vi "Reference Imaging Source.vi"() -> ()   [LabVIEW 2014]
uses:
  <vilib>/userdefined/High Color/IMAQdx.ctl
  <vilib>/vision/driver/IMAQdx.llb/IMAQdx Buffer Number Mode.ctl
  <vilib>/vision/driver/NI_Vision_Acquisition_Software.lvlib
  <resource>/objmgr/imaqdx.rc
panel:
  out "Ref Path":path
  out "Init Message":string
  out "Device Serial Number":string
  out "Success?":bool
  out "error out  - closing camera":errorcluster
  out "Message":string
  out "Warning":bool
  in  "Overwrite?":bool
  in  "Exposure Time µs":dbl=50.0 min=50.0 max=2000000.0 step=1.0 format="%#_8f"
  out "Buffer Number Out":u32
  in  "Nom Ref":string="ref"
  in  "File Path (for Snap! function)":path
  in  "snap":bool
  in  "Gain (dB)":dbl=18.06 min=0.0 max=18.06 step=0.1
  in  "File to ref":bool
  in  "Ref To File":bool
  in  "End Point 2":cluster{"X":i32, "Y":i32}
  in  "Start Point 2":cluster{"X":i32, "Y":i32}
  in  "End Point 1":cluster{"X":i32, "Y":i32}
  in  "Start Point 1":cluster{"X":i32, "Y":i32}
  out "error out":errorcluster
  in  "error in (no error)":errorcluster
  in  "Rectangle d'encardrement":T1
  in  "ref":bool
  out "Coordonnées":i32[](array[numeric])
  in  "stop":bool
  out "Image":T2(plugin-control)
  in  "Session":T3="cam0"
  # "Références Champs Proches/Champs Lointains"
  # "Utiliser outil OVALE pour effectuer la sélection"
  # "Beta version :)"
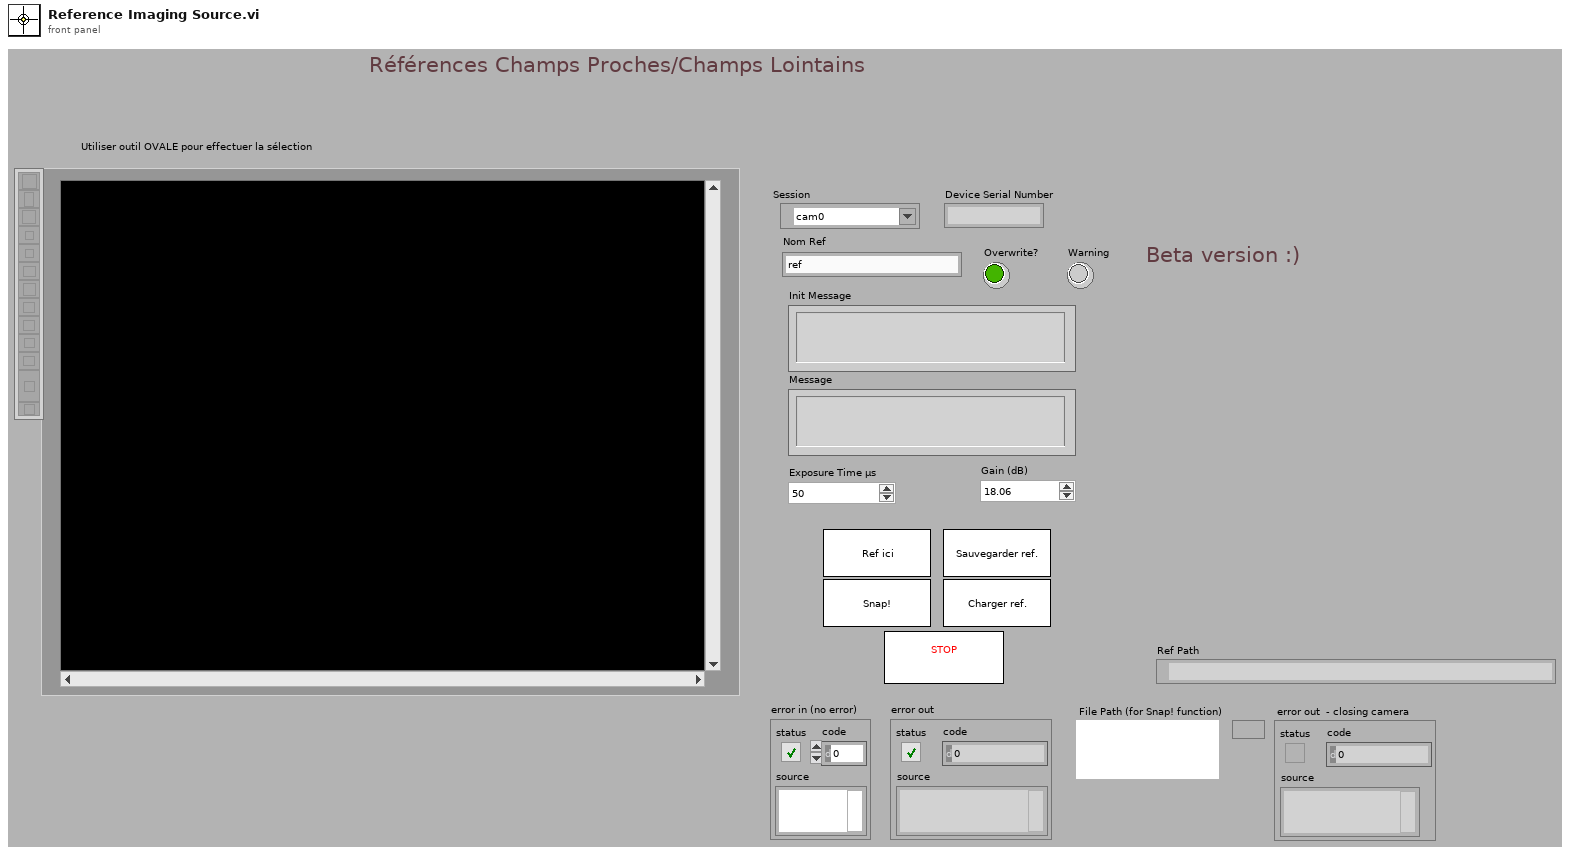
[diagram p1: front panel]
types:
  T1 = cluster{"Left":i32, "Top":i32, "Right":i32, "Bottom":i32}
  T2 = typedef "IMAQ Image.ctl" = refnum<image>
  T3 = typedef "IMAQdx.ctl" = refnum<k21>
  T4 = enum16{"open", "replace", "create", "open or create", "replace or create", "replace or create with confirmation"}
  T5 = typedef "NI_Vision_Acquisition_Software.lvlib/IMAQdx Buffer Number Mode.ctl" = enum32{"Next", "Last", "Buffer Number"}
  T6 = enum8{"Enabled", "Disabled", "Disabled and Grayed Out"}
  T7 = typedef "Image Type" = u32
  T8 = cluster{"Start Point 1":cluster{"X":i32, "Y":i32}, "End Point 1":cluster{"X":i32, "Y":i32}, "Start Point 2":cluster{"X":i32, "Y":i32}, "End Point 2":cluster{"X":i32, "Y":i32}}
  T9 = enum32{"invalid app kind", "Development System", "Run Time System", "Student Edition", "Embedded LabVIEW", "Evaluation", "Custom"}
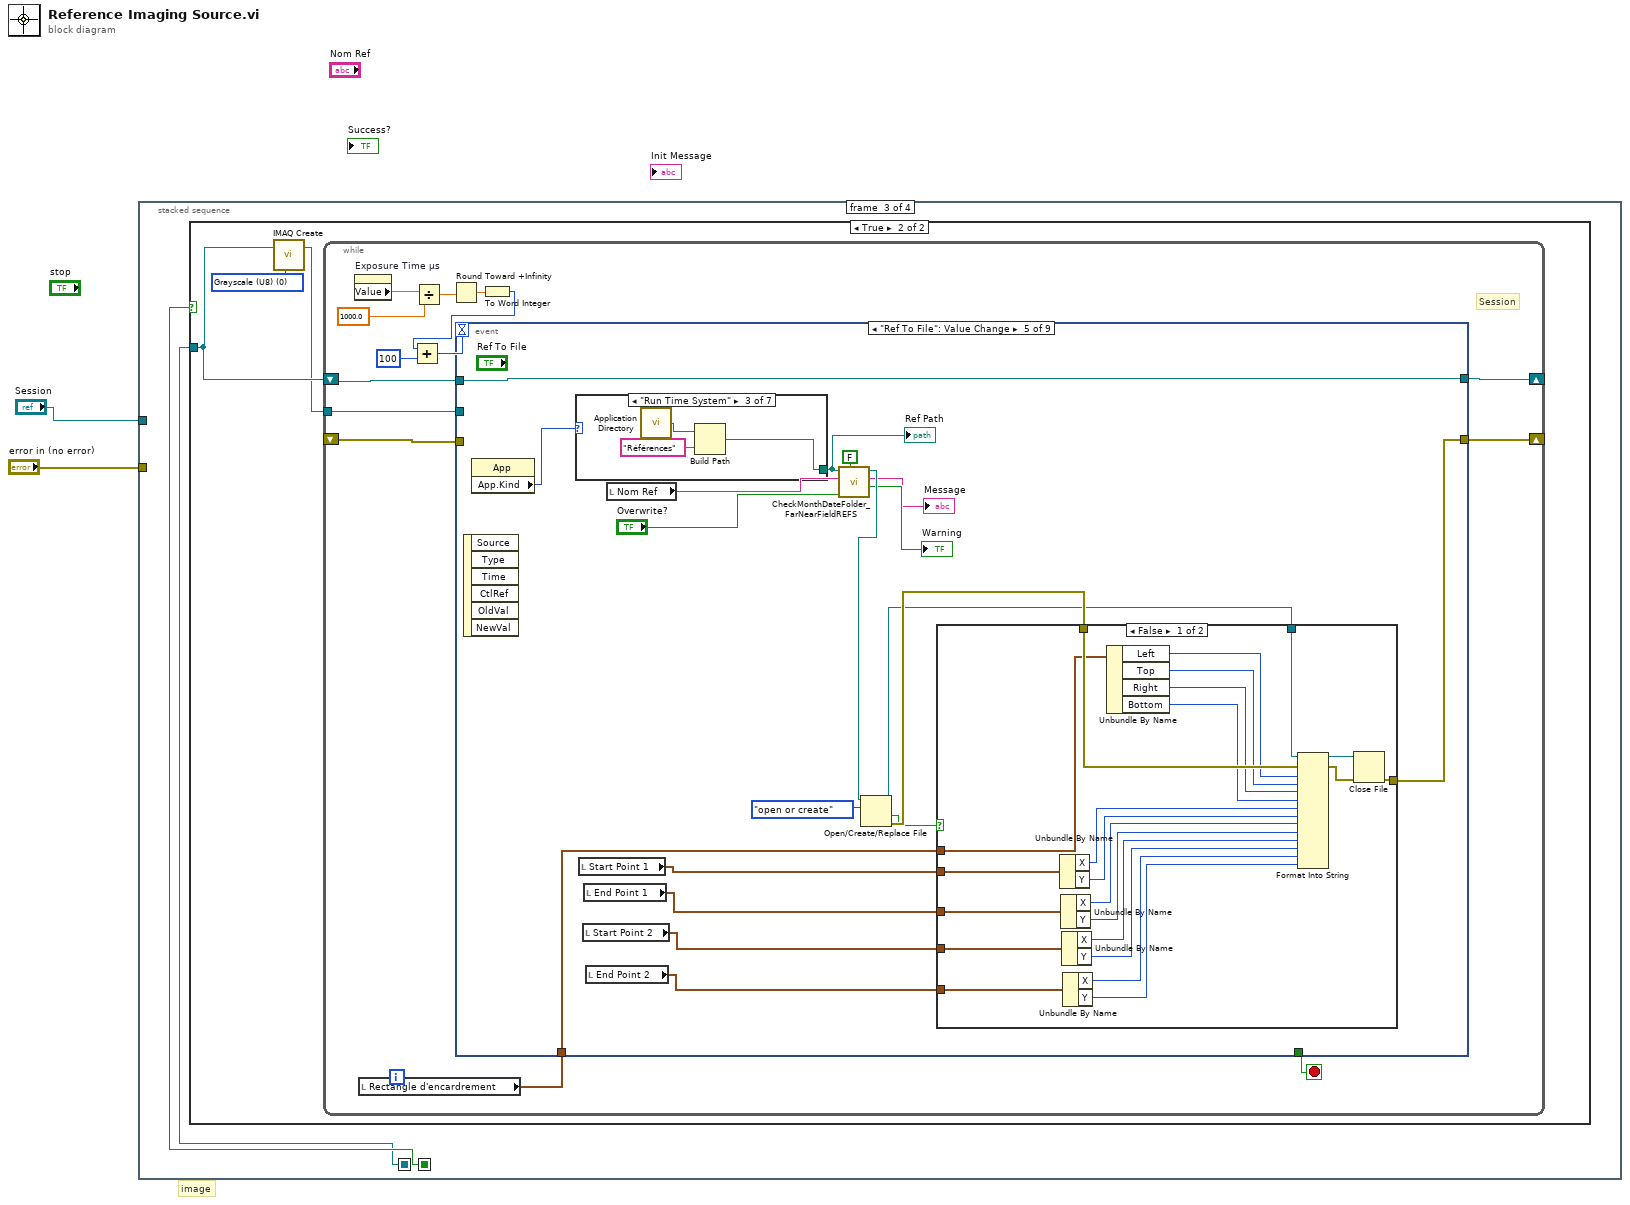
[diagram p0: block diagram]
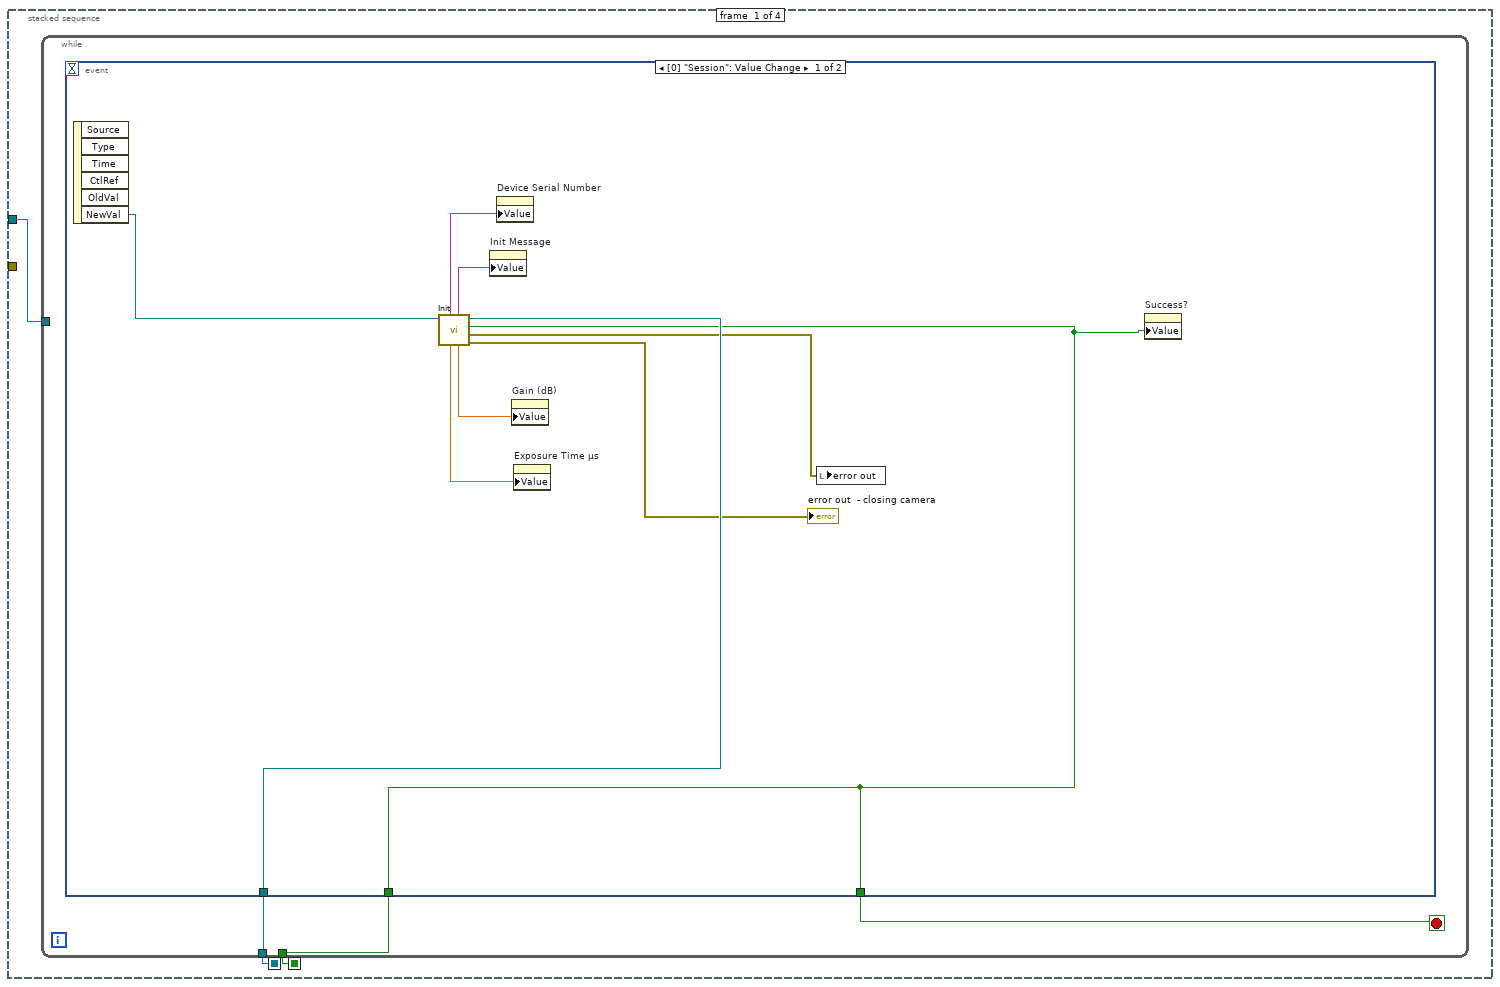
[diagram p2: hidden frame]
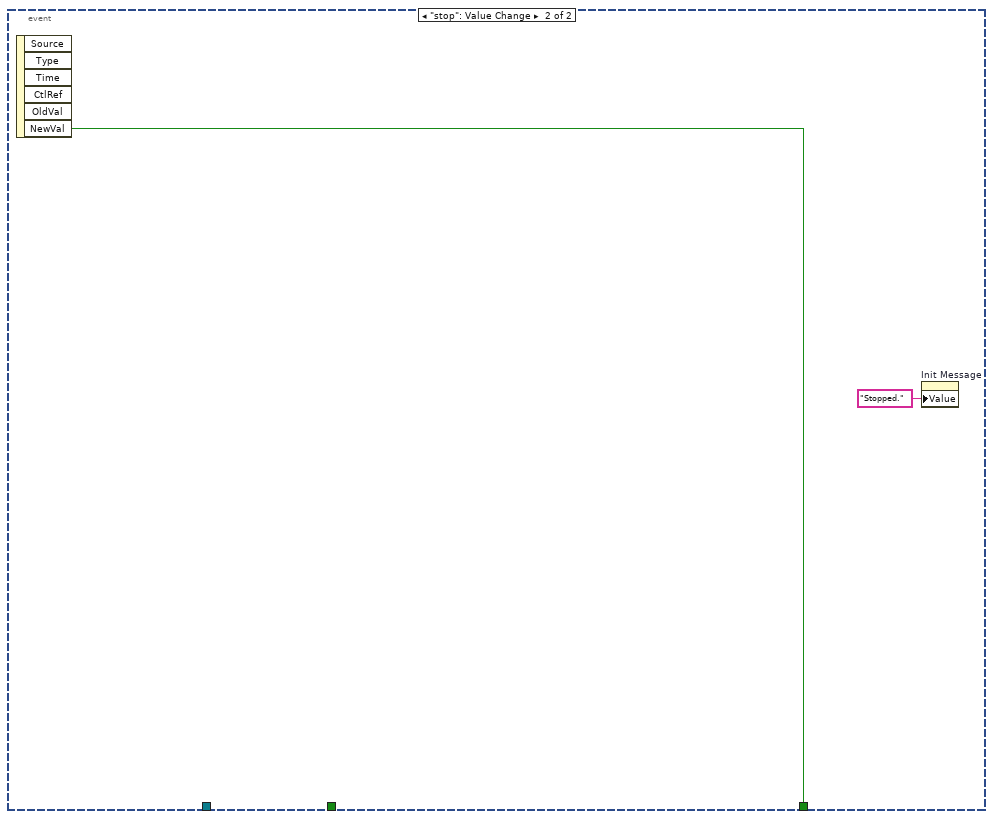
[diagram p3: hidden frame]
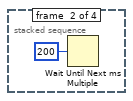
[diagram p4: hidden frame]
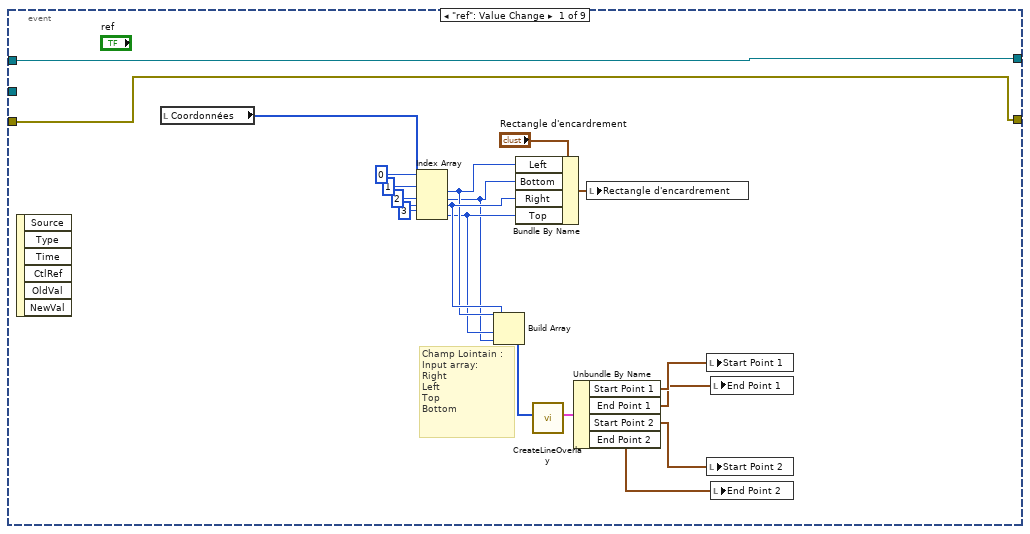
[diagram p6: hidden frame]
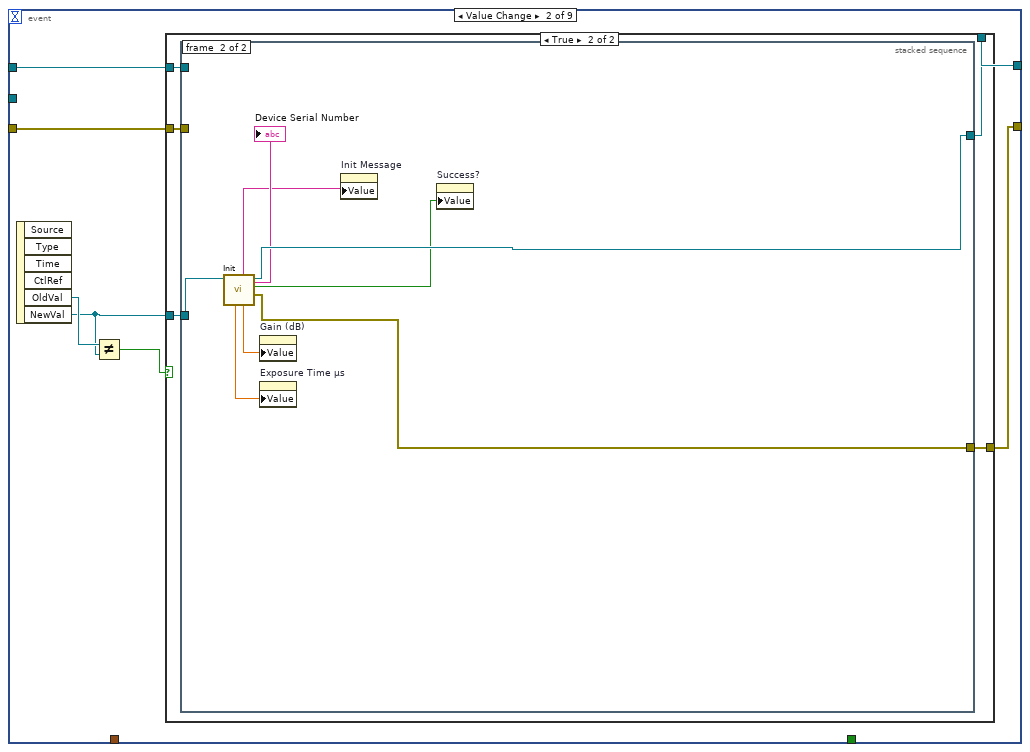
[diagram p7: hidden frame]
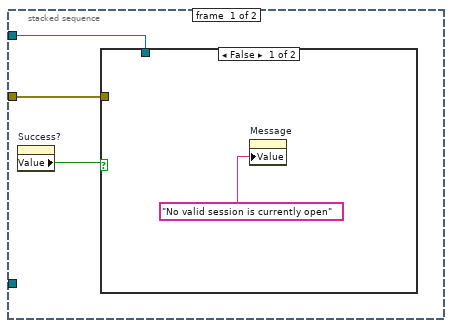
[diagram p9: hidden frame]
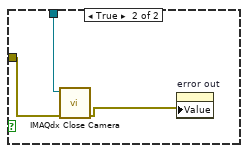
[diagram p10: hidden frame]
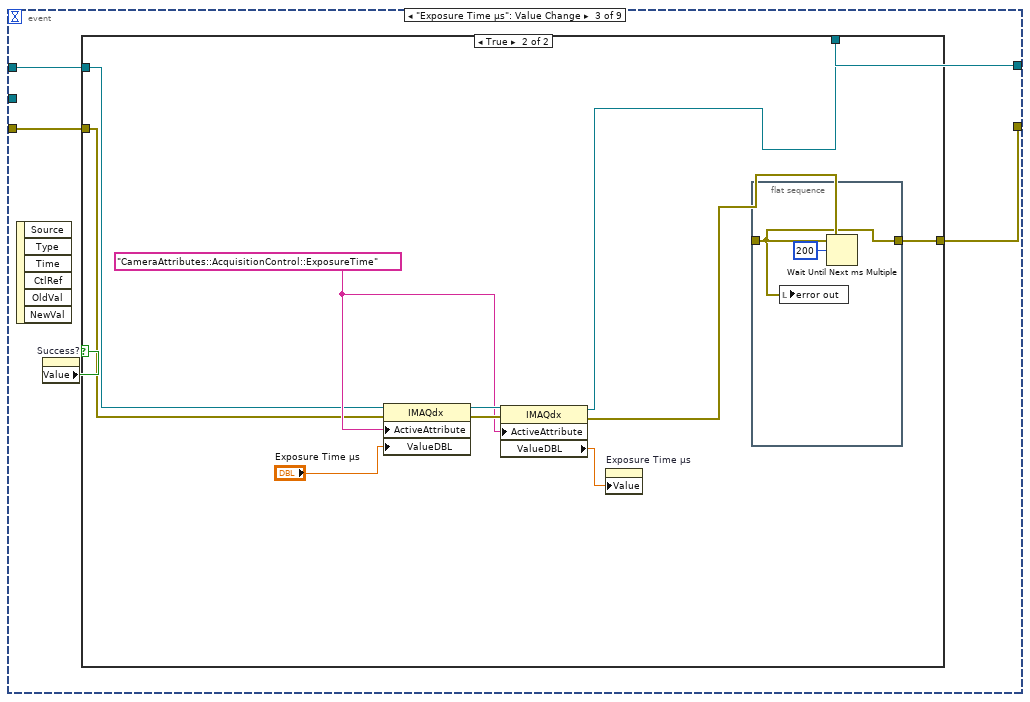
[diagram p11: hidden frame]
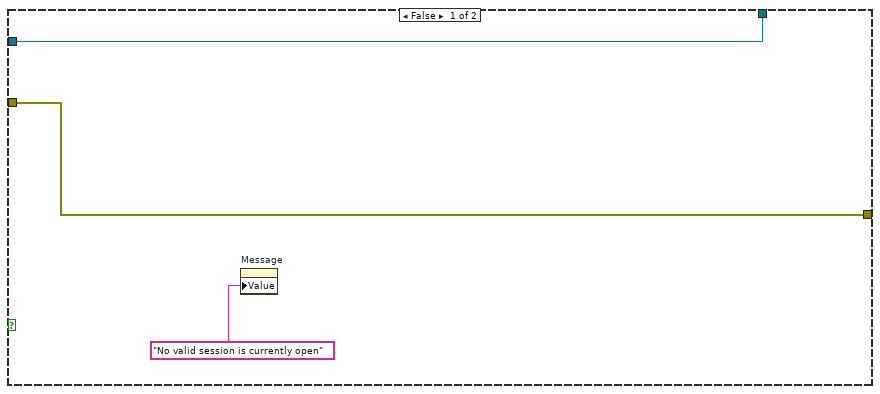
[diagram p12: hidden frame]
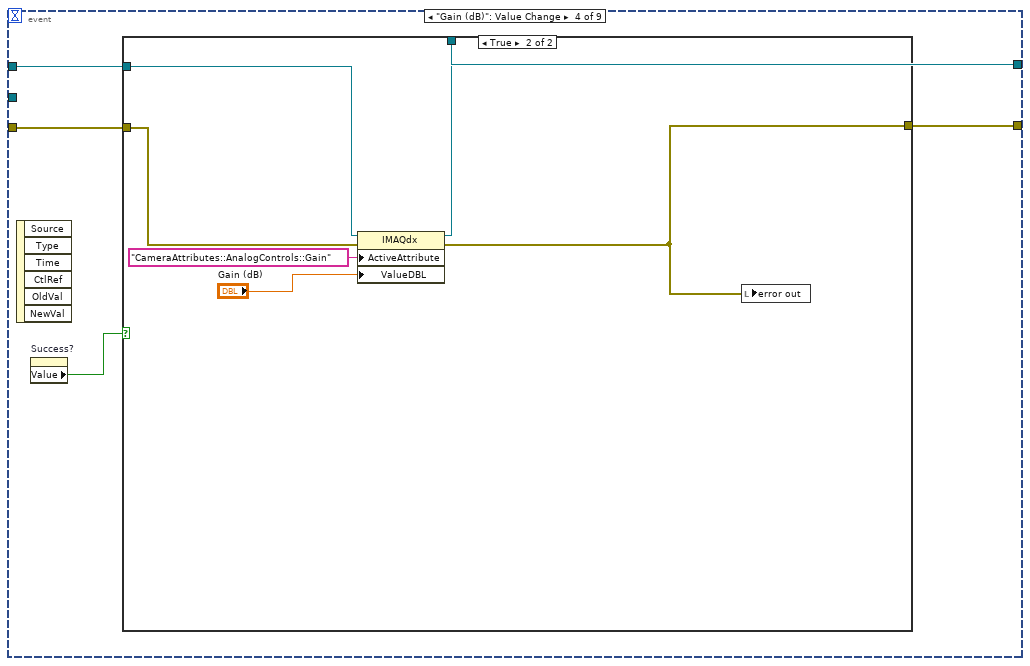
[diagram p13: hidden frame]
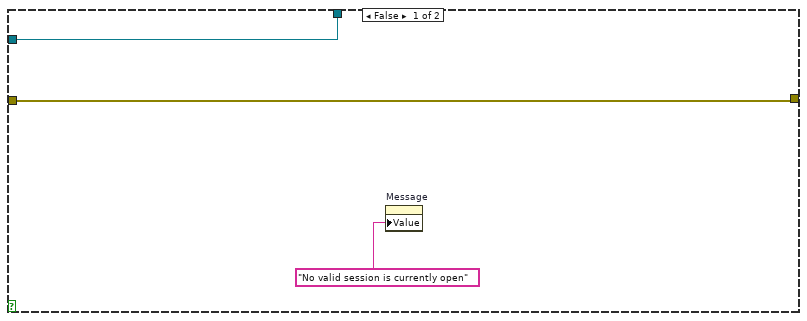
[diagram p14: hidden frame]
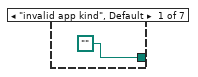
[diagram p15: hidden frame]
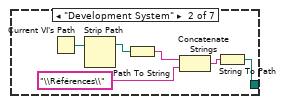
[diagram p16: hidden frame]
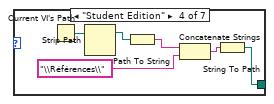
[diagram p17: hidden frame]
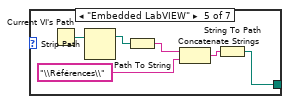
[diagram p18: hidden frame]
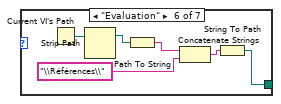
[diagram p19: hidden frame]
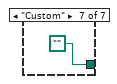
[diagram p20: hidden frame]
diagram:
  # "image"
  n1 = stacked-sequence {
    seq-local: [w4 _ _ _] -> [_ _ w21 _]
    seq-local: [w3 _ _ _] -> [_ _ w22 _]
    tunnel: "Session" -> [w5 _ _ _]
    tunnel: "error in (no error)" -> [_ _ _ _]
    frame #0 {
      n2 = while {
        tunnel: w5 -> [_]
        tunnel: [w7] -> w4
        tunnel: [w6] -> w3
        stop <- w8 stop-if-true
        n3 = event shown="[0] \"Session\": Value Change" {
          selector: _ -> [_ _]
          dyn-events: _ -> [_ _]
          timeout: _ -> [_ _]
          tunnel: [w9 w19] -> w8
          tunnel: [w17 _] -> w7
          tunnel: [w9 _] -> w6
          event Value Change {
            n4 = event-data() -> ("NewVal"=w16:T3)  [unwired: 1 in, 5 out]
            n5 = call "Init.vi"("Session"=w16) -> ("error out  - closing camera"=→"error out  - closing camera":errorcluster, "error out"=w13:errorcluster, "Success?"=w9:bool, "IMAQdx Session OUT"=w17:T3, "Gain - READ"=w15:dbl, "Message"=w11:string, "Exposure Time - READ"=w14:dbl, "Device Serial Number"=w10:string)  [unwired: 3 in]
            n6 = property on="Init Message" class="Str"("Value"=w11) -> ()  [unwired: 2 in, 2 out]
            n7 = property on="Device Serial Number" class="Str"("Value"=w10) -> ()  [unwired: 2 in, 2 out]
            n8 = property on="Gain (dB)" class="DigNum (strict)"("Value"=w15) -> ()  [unwired: 2 in, 2 out]
            n9 = property on="Exposure Time µs" class="DigNum (strict)"("Value"=w14) -> ()  [unwired: 2 in, 2 out]
            n10 = local write "error out"(w13) -> ()
            n11 = property on="Success?" class="Bool (strict)"("Value"=w9) -> ()  [unwired: 2 in, 2 out]
          }
          event "stop": Value Change {
            n12 = event-data() -> ("NewVal"=w19:bool)  [unwired: 1 in, 5 out]
            n13 = property on="Init Message" class="Str"("Value"="Stopped." ("Init Message")) -> ()  [unwired: 2 in, 2 out]
          }
        }
      }
    }
    frame #1 {
      n14 = Wait Until Next ms Multiple(millisecond multiple=u32 200) -> ()  [unwired: 1 out]
    }
    frame #2 {
      n15 = case shown="True" w22 {
        tunnel: w21 -> [_ w24]
        frame False {
        }
        frame True {
          w25 = T7 0 items=["Grayscale (U8)", "Grayscale (I16)", "Grayscale (SGL)", "Complex (CSG)", "RGB (U32)", "HSL (U32)", "RGB (U64)", "Grayscale (U16)"] ("Image Type")
          n16 = call "IMAQ Create"("Image Name"=w24, "Image Type"=w25) -> ("New Image"=w23:T2)  [unwired: 2 in, 2 out]
          n17 = while {
            shift-right: [w37] -> _
            shift-left: _ -> [w38]
            shift-right: [w35] -> _
            shift-left: w24 -> [w36]
            tunnel: w23 -> [w26]
            stop <- w39 stop-if-true
            # "Session"
            n18 = property on="Exposure Time µs" class="DigNum (strict)"() -> ("Value"=w27:dbl)  [unwired: 2 in, 2 out]
            n19 = local read "Rectangle d'encardrement"() -> (w28:T1)
            n20 = Divide(x=w27, y=1000.0) -> (x/y=w30:dbl)
            n21 = Round Toward +Infinity(x=w30) -> (ceil(x): smallest int >= x=w32:dbl)
            n22 = To Word Integer(number=w32) -> (16bit integer=w29:i16)
            n23 = Add(x=w29, y=i16 100) -> (x+y=w33:i16)
            n24 = event shown="[4] \"Ref To File\": Value Change" {
              selector: _ -> [_ _ _ _ _ _ _ _ _]
              dyn-events: _ -> [_ _ _ _ _ _ _ _ _]
              timeout: w33 -> [_ _ _ _ _ _ _ _ _]
              tunnel: [_ _ _ _ _ _ _ w254 _] -> w39
              tunnel: w38 -> [w40 w65 w90 w112 _ w203 w238 w255 w268]
              tunnel: [w40 w63 w92 w109 w136 w198 w239 _ w267] -> w37
              tunnel: w36 -> [w41 w62 w91 w111 w124 w197 w237 w256 w266]
              tunnel: [w41 w64 w89 w110 w124 w197 w236 _ w265] -> w35
              tunnel: w28 -> [_ _ _ _ w135 _ _ _ _]
              tunnel: w26 -> [_ _ _ _ _ _ w235 _ w260]
              event "ref": Value Change {
                # "Champ Lointain :\nInput array:\nRight\nLeft\nTop\nBottom"
                n25 = event-data() -> ()  [unwired: 1 in, 6 out]
                n26 = local read "Coordonnées"() -> (w52:i32[])
                n27 = Index Array(array=w52, index #1=0 ("index"), index #2=1 ("index"), index #3=2 ("index"), index #4=3 ("index")) -> (element #1=w45:i32, element #2=w43:i32, element #3=w46:i32, element #4=w44:i32)
                n28 = Build Array(w46, w45, w44, w43) -> (w42:i32[])
                n29 = Bundle By Name(cluster="Rectangle d'encardrement", "Left"=w45, "Bottom"=w43, "Right"=w46, "Top"=w44) -> (w53:T1)
                n30 = call "CreateLineOverlay.vi"("Bounding rectangle"=w42) -> ("Lines"=w51:T8)  [unwired: 8 in, 1 out]
                n31 = Unbundle By Name(w51) -> ("Start Point 1"=w50:cluster{"X":i32, "Y":i32}, "End Point 1"=w49:cluster{"X":i32, "Y":i32}, "Start Point 2"=w48:cluster{"X":i32, "Y":i32}, "End Point 2"=w47:cluster{"X":i32, "Y":i32})
                n32 = local write "Rectangle d'encardrement"(w53) -> ()
                n33 = local write "Start Point 1"(w50) -> ()
                n34 = local write "Start Point 2"(w48) -> ()
                n35 = local write "End Point 1"(w49) -> ()
                n36 = local write "End Point 2"(w47) -> ()
              }
              event Value Change {
                n37 = event-data() -> ("OldVal"=w60:T3, "NewVal"=w59:T3)  [unwired: 1 in, 4 out]
                n38 = Not Equal?(x=w60, y=w59) -> (x != y?=w61:bool)
                n39 = case shown="True" w61 {
                  tunnel: w65 -> [w66 w72]
                  tunnel: w59 -> [w67 w71]
                  tunnel: [w67 w70] -> w64
                  tunnel: [w66 w69] -> w63
                  tunnel: w62 -> [_ w68]
                  frame False {
                  }
                  frame True {
                    n40 = stacked-sequence {
                      tunnel: w72 -> [w75 _]
                      tunnel: w71 -> [_ w87]
                      tunnel: [_ w84] -> w70
                      tunnel: [_ w82] -> w69
                      tunnel: w68 -> [w74 _]
                      frame #0 {
                        n41 = property on="Success?" class="Bool (strict)"() -> ("Value"=w73:bool)  [unwired: 2 in, 2 out]
                        n42 = case shown="False" w73 {
                          tunnel: w75 -> [_ w79]
                          tunnel: w74 -> [_ w77]
                          frame False {
                            n43 = property on="Message" class="Str"("Value"="No valid session is currently open" ("Message")) -> ()  [unwired: 2 in, 2 out]
                          }
                          frame True {
                            n44 = call <vilib>:"IMAQdx Close Camera.vi"("error in"=w79, "Session In"=w77) -> ("error out"=w78:errorcluster)  [unwired: 9 in]
                            n45 = property on="error out" class="Clust (strict)"("Value"=w78) -> ()  [unwired: 2 in, 2 out]
                          }
                        }
                      }
                      frame #1 {
                        n46 = call "Init.vi"("Session"=w87) -> ("error out"=w82:errorcluster, "Success?"=w83:bool, "IMAQdx Session OUT"=w84:T3, "Gain - READ"=w86:dbl, "Message"=w80:string, "Exposure Time - READ"=w85:dbl, "Device Serial Number"=→"Device Serial Number":string)  [unwired: 3 in, 1 out]
                        n47 = property on="Gain (dB)" class="DigNum (strict)"("Value"=w86) -> ()  [unwired: 2 in, 2 out]
                        n48 = property on="Exposure Time µs" class="DigNum (strict)"("Value"=w85) -> ()  [unwired: 2 in, 2 out]
                        n49 = property on="Init Message" class="Str"("Value"=w80) -> ()  [unwired: 2 in, 2 out]
                        n50 = property on="Success?" class="Bool (strict)"("Value"=w83) -> ()  [unwired: 2 in, 2 out]
                      }
                    }
                  }
                }
              }
              event "Exposure Time µs": Value Change {
                n51 = event-data() -> ()  [unwired: 1 in, 6 out]
                n52 = property on="Success?" class="Bool (strict)"() -> ("Value"=w88:bool)  [unwired: 2 in, 2 out]
                n53 = case shown="True" w88 {
                  tunnel: [w94 w104] -> w92
                  tunnel: w91 -> [w95 w96]
                  tunnel: w90 -> [w94 w97]
                  tunnel: [w95 w101] -> w89
                  frame False {
                    n54 = property on="Message" class="Str"("Value"="No valid session is currently open" ("Message")) -> ()  [unwired: 2 in, 2 out]
                  }
                  frame True {
                    w98 = "CameraAttributes::AcquisitionControl::ExposureTime" ("ActiveAttribute")
                    n55 = property class="IMAQdx"(reference=w96, error in=w97, "ActiveAttribute"=w98, "ValueDBL"="Exposure Time µs") -> (reference out=w103:T3, error out=w102:errorcluster)
                    n56 = property class="IMAQdx"(reference=w103, error in=w102, "ActiveAttribute"=w98) -> (reference out=w101:T3, error out=w100:errorcluster, "ValueDBL"=w99:dbl)
                    n57 = property on="Exposure Time µs" class="DigNum (strict)"("Value"=w99) -> ()  [unwired: 2 in, 2 out]
                    n58 = flat-sequence {
                      tunnel: w100 -> [w106]
                      tunnel: [w106] -> w104
                      frame #0 {
                        n59 = local write "error out"(w106) -> ()
                        n60 = Wait Until Next ms Multiple(millisecond multiple=u32 200) -> ()  [unwired: 1 out]
                      }
                    }
                  }
                }
              }
              event "Gain (dB)": Value Change {
                n61 = event-data() -> ()  [unwired: 1 in, 6 out]
                n62 = property on="Success?" class="Bool (strict)"() -> ("Value"=w108:bool)  [unwired: 2 in, 2 out]
                n63 = case shown="True" w108 {
                  tunnel: w112 -> [w115 w121]
                  tunnel: w111 -> [w114 w118]
                  tunnel: [w114 w117] -> w110
                  tunnel: [w115 w116] -> w109
                  frame False {
                    n64 = property on="Message" class="Str"("Value"="No valid session is currently open" ("Message")) -> ()  [unwired: 2 in, 2 out]
                  }
                  frame True {
                    n65 = property class="IMAQdx"(reference=w118, error in=w121, "ActiveAttribute"="CameraAttributes::AnalogControls::Gain", "ValueDBL"="Gain (dB)") -> (reference out=w117:T3, error out=w116:errorcluster)
                    n66 = local write "error out"(w116) -> ()
                  }
                }
              }
              event "Ref To File": Value Change {
                n67 = event-data() -> ()  [unwired: 1 in, 6 out]
                n68 = property class="App"() -> ("App.Kind"=w123:T9)  [unwired: 2 in, 2 out]
                n69 = case shown="\"Run Time System\"" w123 {
                  tunnel: [path "" w142 w148 w151 w157 w163 path ""] -> w130
                  frame "invalid app kind", Default {
                  }
                  frame "Development System" {
                    n70 = Current VI's Path() -> (path=w147:path)
                    n71 = Strip Path(path=w147) -> (stripped path=w146:path)  [unwired: 1 out]
                    n72 = Path To String(path=w146) -> (string=w145:string)
                    n73 = Concatenate Strings(w145, "\\Références\\") -> (w143:string)
                    n74 = String To Path(string=w143) -> (path=w142:path)
                  }
                  frame "Run Time System" {
                    n75 = call <vilib>:"Application Directory.vi"() -> ("Application Directory"=w150:path)
                    n76 = Build Path(base path=w150, name or relative path="Références") -> (appended path=w148:path)
                  }
                  frame "Student Edition" {
                    n77 = Current VI's Path() -> (path=w156:path)
                    n78 = Strip Path(path=w156) -> (stripped path=w155:path)  [unwired: 1 out]
                    n79 = Path To String(path=w155) -> (string=w154:string)
                    n80 = Concatenate Strings(w154, "\\Références\\") -> (w152:string)
                    n81 = String To Path(string=w152) -> (path=w151:path)
                  }
                  frame "Embedded LabVIEW" {
                    n82 = Current VI's Path() -> (path=w162:path)
                    n83 = Strip Path(path=w162) -> (stripped path=w161:path)  [unwired: 1 out]
                    n84 = Path To String(path=w161) -> (string=w160:string)
                    n85 = Concatenate Strings(w160, "\\Références\\") -> (w158:string)
                    n86 = String To Path(string=w158) -> (path=w157:path)
                  }
                  frame "Evaluation" {
                    n87 = Current VI's Path() -> (path=w168:path)
                    n88 = Strip Path(path=w168) -> (stripped path=w167:path)  [unwired: 1 out]
                    n89 = Path To String(path=w167) -> (string=w166:string)
                    n90 = Concatenate Strings(w166, "\\Références\\") -> (w164:string)
                    n91 = String To Path(string=w164) -> (path=w163:path)
                  }
                  frame "Custom" {
                  }
                }
                "Ref Path" <- w130
                n92 = local read "Start Point 1"() -> (w134:cluster{"X":i32, "Y":i32})
                n93 = local read "Start Point 2"() -> (w132:cluster{"X":i32, "Y":i32})
                n94 = local read "End Point 1"() -> (w133:cluster{"X":i32, "Y":i32})
                n95 = local read "End Point 2"() -> (w131:cluster{"X":i32, "Y":i32})
                n96 = local read "Nom Ref"() -> (w129:string)
                n97 = call "CheckMonthDateFolder_FarNearFieldREFS.vi"("Folder Path Control"=w130, "File Name"=w129, "Overwrite?"="Overwrite?", "Automatic date folder nesting?"=FALSE) -> ("File Path"=w127:path, "Message"=→"Message":string, "Warning"=→"Warning":bool)  [unwired: 4 in]
                n98 = Open/Create/Replace File(file path (use dialog)=w127, operation (0:open)=T4."open or create") -> (refnum out=w138:refnum<file>, cancelled=w137:bool, error out=w139:errorcluster)  [unwired: 4 in]
                n99 = case shown="False" w137 {
                  tunnel: w139 -> [w191 w196]
                  tunnel: w138 -> [w189 _]
                  tunnel: [w175 w192] -> w136
                  tunnel: w135 -> [w174 _]
                  tunnel: w134 -> [w173 _]
                  tunnel: w133 -> [w172 _]
                  tunnel: w132 -> [w171 _]
                  tunnel: w131 -> [w170 _]
                  frame False {
                    n100 = Unbundle By Name(w173) -> ("X"=w185:i32, "Y"=w184:i32)
                    n101 = Unbundle By Name(w172) -> ("X"=w183:i32, "Y"=w182:i32)
                    n102 = Unbundle By Name(w171) -> ("X"=w181:i32, "Y"=w180:i32)
                    n103 = Unbundle By Name(w170) -> ("X"=w179:i32, "Y"=w178:i32)
                    n104 = Unbundle By Name(w174) -> ("Left"=w190:i32, "Top"=w188:i32, "Right"=w187:i32, "Bottom"=w186:i32)
                    n105 = Format Into String(initial string=w189, error in=w191, w190, w188, w187, w186, w185, w184, w183, w182, w181, w180, w179, w178) -> (resulting string=w177:refnum<file>, error out=w176:errorcluster)  [unwired: 1 in]
                    n106 = Close File(refnum=w177, error in=w176) -> (error out=w175:errorcluster)  [unwired: 1 out]
                  }
                  frame True {
                    n107 = Bundle By Name(cluster=w196, "status"=FALSE, "code"=0, "source"="") -> (w192:errorcluster)
                  }
                }
              }
              event "File to ref": Value Change {
                n108 = event-data() -> ()  [unwired: 1 in, 6 out]
                n109 = Open/Create/Replace File(error in=w203, prompt="Fichier à charger", access (0:read/write)=enum16{"read/write", "read-only", "write-only"}."read-only") -> (refnum out=w200:refnum<file>, cancelled=w199:bool, error out=w202:errorcluster)  [unwired: 3 in]
                n110 = case shown="False" w199 {
                  tunnel: w202 -> [w208 _]
                  tunnel: w200 -> [w231 _]
                  tunnel: [w205 errorcluster {"status"=FALSE, "code"=0, "source"=""} ("error out")] -> w198
                  frame False {
                    n111 = Scan From String("%d %d %d %d %d %d %d %d %d %d %d %d" ("format string"), w231, w208) -> (w207:refnum<file>, w206:errorcluster, output 1=w228:i32, output 2=w227:i32, output 3=w226:i32, output 4=w225:i32, output 5=w223:i32, output 6=w222:i32, output 7=w218:i32, output 8=w217:i32, output 9=w214:i32, output 10=w213:i32, output 11=w210:i32, output 12=w209:i32)  [unwired: 12 in]
                    n112 = local read "Rectangle d'encardrement"() -> (w230:T1)
                    n113 = local read "Start Point 2"() -> (w216:cluster{"X":i32, "Y":i32})
                    n114 = local read "End Point 2"() -> (w212:cluster{"X":i32, "Y":i32})
                    n115 = local read "Start Point 1"() -> (w224:cluster{"X":i32, "Y":i32})
                    n116 = local read "End Point 1"() -> (w220:cluster{"X":i32, "Y":i32})
                    n117 = Bundle By Name(cluster=w224, "X"=w223, "Y"=w222) -> (w221:cluster{"X":i32, "Y":i32})
                    n118 = Bundle By Name(cluster=w220, "X"=w218, "Y"=w217) -> (w219:cluster{"X":i32, "Y":i32})
                    n119 = Bundle By Name(cluster=w230, "Left"=w228, "Top"=w227, "Right"=w226, "Bottom"=w225) -> (w229:T1)
                    n120 = Bundle By Name(cluster=w212, "X"=w210, "Y"=w209) -> (w211:cluster{"X":i32, "Y":i32})
                    n121 = Bundle By Name(cluster=w216, "X"=w214, "Y"=w213) -> (w215:cluster{"X":i32, "Y":i32})
                    n122 = local write "Start Point 1"(w221) -> ()
                    n123 = local write "End Point 1"(w219) -> ()
                    n124 = local write "Start Point 2"(w215) -> ()
                    n125 = local write "End Point 2"(w211) -> ()
                    n126 = local write "Rectangle d'encardrement"(w229) -> ()
                    n127 = Close File(refnum=w207, error in=w206) -> (error out=w205:errorcluster)  [unwired: 1 out]
                  }
                  frame True {
                  }
                }
              }
              event "snap": Value Change {
                n128 = event-data() -> ()  [unwired: 1 in, 6 out]
                n129 = property on="Success?" class="Bool (strict)"() -> ("Value"=w234:bool)  [unwired: 2 in, 2 out]
                n130 = case shown="False" w234 {
                  tunnel: [w240 w251] -> w239
                  tunnel: w238 -> [w240 w249]
                  tunnel: w237 -> [w241 w245]
                  tunnel: [w241 w244] -> w236
                  tunnel: w235 -> [_ w243]
                  frame False {
                    n131 = property on="Message" class="Str"("Value"="No valid session is currently open" ("Message")) -> ()  [unwired: 2 in, 2 out]
                  }
                  frame True {
                    n132 = call <vilib>:"IMAQdx Get Image.vi"("Buffer Number Mode (Next)"=IMAQdx_Buffer_Number_Mode."Buffer Number", "error in"=w249, "Image In"=w243, "Session In"=w245) -> ("error out"=w248:errorcluster, "Image Out"=w247:T2, "Session Out"=w244:T3)  [unwired: 4 in, 1 out]
                    n133 = call-poly "IMAQ Write File 2"("error in (no error)"=w248, "File Path"="File Path (for Snap! function)", "Image"=w247) -> ("error out"=w251:errorcluster)  [unwired: 7 in, 1 out]
                  }
                }
              }
              event "stop": Value Change {
                n134 = event-data() -> ("NewVal"=w254:bool)  [unwired: 1 in, 5 out]
                n135 = call <vilib>:"IMAQdx Close Camera.vi"("error in"=w255, "Session In"=w256) -> ("error out"=→"error out":errorcluster)  [unwired: 9 in]
                n136 = property on="Session" class="IMAQdx (strict)"("DisabledEnum"=T6."Enabled" ("Disabled")) -> ()  [unwired: 2 in, 2 out]
                n137 = property on="Init Message" class="Str"("Value"="Stopped." ("Init Message")) -> ()  [unwired: 2 in, 2 out]
                n138 = property on="Message" class="Str"("Value"="" ("Message")) -> ()  [unwired: 2 in, 2 out]
              }
              event Timeout {
                w261 = 5 items=["None", "Selection Tool", "Point Tool", "Line Tool", "Rectangle Tool", "Oval Tool", "Polygon Tool", "ClosedFreehandTool", "Annulus Tool", "Rotated Rectangle Tool", "Zoom Tool", "Pan Tool", "Polyline Tool", "Freehand Tool"] ("Tool")
                n139 = event-data() -> ()  [unwired: 1 in, 3 out]
                n140 = property on="Success?" class="Bool (strict)"() -> ("Value"=w259:bool)  [unwired: 2 in, 2 out]
                n141 = case shown="True" w259 {
                  tunnel: w268 -> [w270 w292]
                  tunnel: [w270 w291] -> w267
                  tunnel: w266 -> [w271 w290]
                  tunnel: [w271 w289] -> w265
                  tunnel: w260 -> [_ w274]
                  frame False {
                    n142 = property on="Message" class="Str"("Value"="No valid session is currently open" ("Message")) -> ()  [unwired: 2 in, 2 out]
                  }
                  frame True {
                    n143 = property on="Message" class="Str"("Value"="Running..." ("Message")) -> ()  [unwired: 2 in, 2 out]
                    n144 = call <vilib>:"IMAQdx Get Image.vi"("Buffer Number Mode (Next)"=IMAQdx_Buffer_Number_Mode."Buffer Number", "error in"=w292, "Image In"=w274, "Session In"=w290) -> ("error out"=w272:errorcluster, "Buffer Number Out"=→"Buffer Number Out":u32, "Image Out"=w276:T2, "Session Out"=w289:T3)  [unwired: 4 in]
                    n145 = local read "Rectangle d'encardrement"() -> (w286:T1)
                    n146 = call "IMAQ Overlay Oval"("Color"=u32 16716404, "error in (no error)"=w272, "Bounding Rectangle"=w286, "Image"=w276) -> ("error out"=w278:errorcluster, "Image Out"=w284:T2)  [unwired: 6 in]
                    n147 = call "IMAQ Overlay Line"("error in (no error)"=w278, "End Point"="End Point 1", "Start Point"="Start Point 1", "Image"=w284) -> ("error out"=w285:errorcluster, "Image Out"=w283:T2)  [unwired: 6 in]
                    n148 = call "IMAQ Overlay Line"("error in (no error)"=w285, "End Point"="End Point 2", "Start Point"="Start Point 2", "Image"=w283) -> ("error out"=w291:errorcluster, "Image Out"=→"Image":T2)  [unwired: 6 in]
                    n149 = call "IMAQ ImageToArray"("Image"=w276) -> ()  [unwired: 3 in, 5 out]
                    n150 = local write "error out"(w291) -> ()
                  }
                }
                n151 = invoke on="Image" class="ImageControl" method="Get Last Event"() -> ("Tool"=w262:i32, "Coordinates"=w263:i32[])  [unwired: 8 in, 6 out]
                n152 = Equal?(x=w261, y=w262) -> (x = y?=w264:bool)
                n153 = case shown="False" w264 {
                  tunnel: w263 -> [_ w293]
                  frame False {
                  }
                  frame True {
                    "Coordonnées" <- w293
                  }
                }
              }
            }
          }
        }
      }
    }
    frame #3 {
      n154 = property on="stop" class="Bool (strict)"("Value"=FALSE ("stop")) -> ()  [unwired: 2 in, 2 out]
    }
  }
